vi "Ej_14_Histeresis.vi"() -> ()   [LabVIEW 2020]
panel:
  in  "x":dbl
  out "Indicador":bool
  out "Dato Actual":dbl
  out "Bandera":bool
  in  "stop":bool
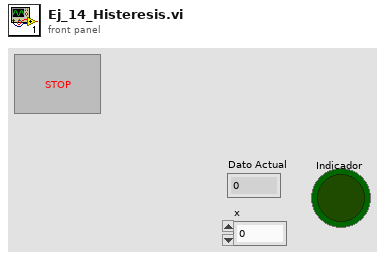
[diagram p1: front panel]
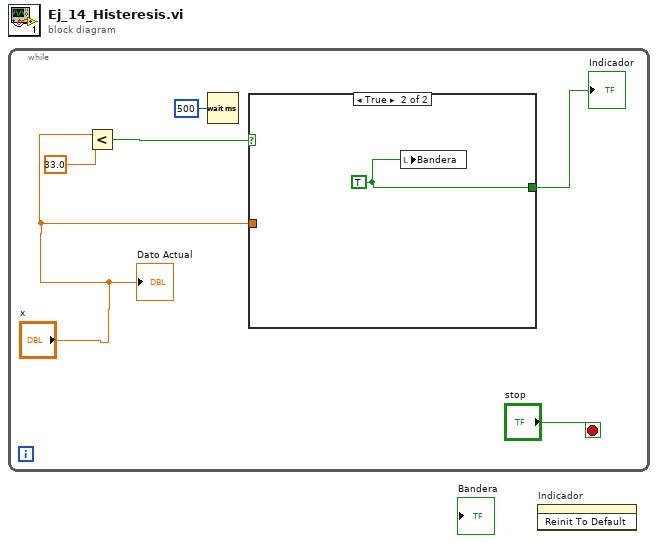
[diagram p0: block diagram]
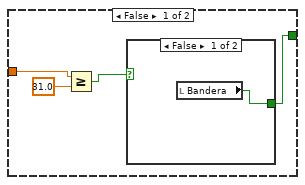
[diagram p2: hidden frame]
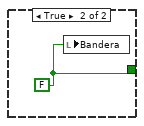
[diagram p3: hidden frame]
diagram:
  n1 = while {
    stop <- "stop" stop-if-true
    n2 = Less?(x="x", y=33.0) -> (x < y?=w3:bool)
    n3 = Wait (ms)(milliseconds to wait=u32 500) -> ()  [unwired: 1 out]
    n4 = case shown="True" w3 {
      tunnel: "x" -> [w10 _]
      tunnel: [w8 w13] -> w2
      frame False {
        n5 = Greater Or Equal?(x=w10, y=31.0) -> (x >= y?=w7:bool)
        n6 = case shown="False" w7 {
          tunnel: [w11 w12] -> w8
          frame False {
            n7 = local read "Bandera"() -> (w11:bool)
          }
          frame True {
            w12 = FALSE
            n8 = local write "Bandera"(w12) -> ()
          }
        }
      }
      frame True {
        w13 = TRUE
        n9 = local write "Bandera"(w13) -> ()
      }
    }
    "Indicador" <- w2
    "Dato Actual" <- "x"
  }
  n10 = invoke on="Indicador" class="Bool (strict)" method="Reinit To Default"() -> ()  [unwired: 3 in, 3 out]
